vi "MASBstat.vi"() -> ()   [LabVIEW 2020]
doc: "Main application front panel."
uses:
  Typedefs/Control and indicators refs.ctl
  Typedefs/EHL state.ctl
  Global variables/VISA resource.vi
  Global variables/Control and indicators refs.vi
  Typedefs/State.ctl
  Typedefs/CV configuration.ctl
panel:
  out "I-V Graph":cluster{"X":dbl, "Y":dbl}[](graph)
  in  "Connect":bool
  in  "Device":refnum<visa-resource-name>
  in  "Measurement":bool
  in  "CV configuration":T1={"E begin (V)"=0.0, "E vertex 1 (V)"=0.0, "E vertex 2 (V)"=0.0, "Cycles"=1, "Scan rate (V/s)"=0.01, "E step (V)"=0.01} {"E step (V)" min=0.01 max=0.25; "Scan rate (V/s)" min=0.01 max=10.0; "Cycles" min=1; "E vertex 2 (V)" min=-3.3 max=3.3; "E vertex 1 (V)" min=-3.3 max=3.3; "E begin (V)" min=-3.3 max=3.3}
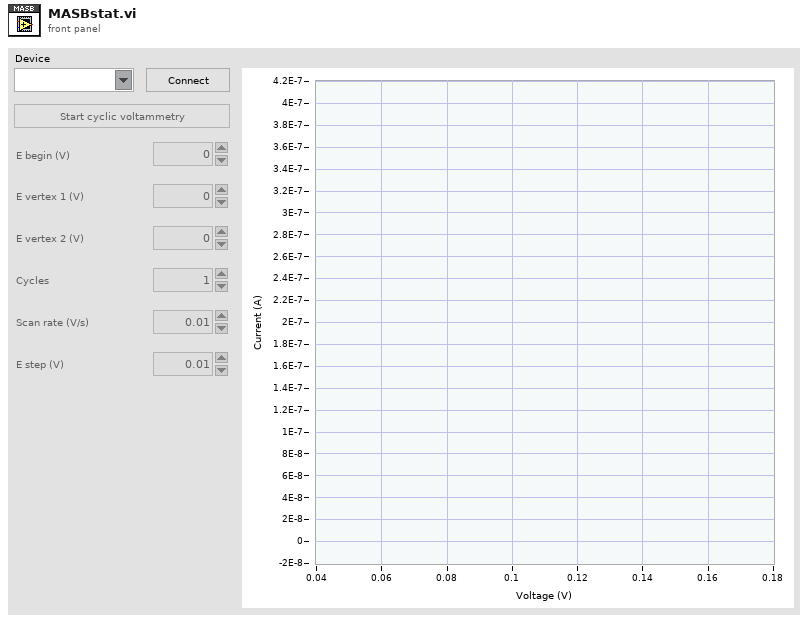
[diagram p1: front panel]
types:
  T1 = typedef "CV configuration.ctl" = cluster{"E begin (V)":dbl, "E vertex 1 (V)":dbl, "E vertex 2 (V)":dbl, "Cycles":u8, "Scan rate (V/s)":dbl, "E step (V)":dbl}
  T2 = typedef "State.ctl" = enum16{"Disconnected", "Connected", "Measuring"}
  T3 = typedef "EHL state.ctl" = cluster{"Semaphore":T4, "Queue":refnum<queue>, "App state":T2}
  T4 = typedef "Semaphore RefNum" = refnum<k1>
  T5 = typedef "Control and indicators refs.ctl" = cluster{"Device":refnum<vi>, "Connect":refnum<vi>, "Measurement":refnum<vi>, "CV configuration":refnum<vi>, "I-V Graph":refnum<vi>}
  T6 = cluster{"E begin (V)":dbl, "E vertex 1 (V)":dbl, "E vertex 2 (V)":dbl, "Cycles":u8, "Scan rate (V/s)":dbl, "E step (V)":dbl}
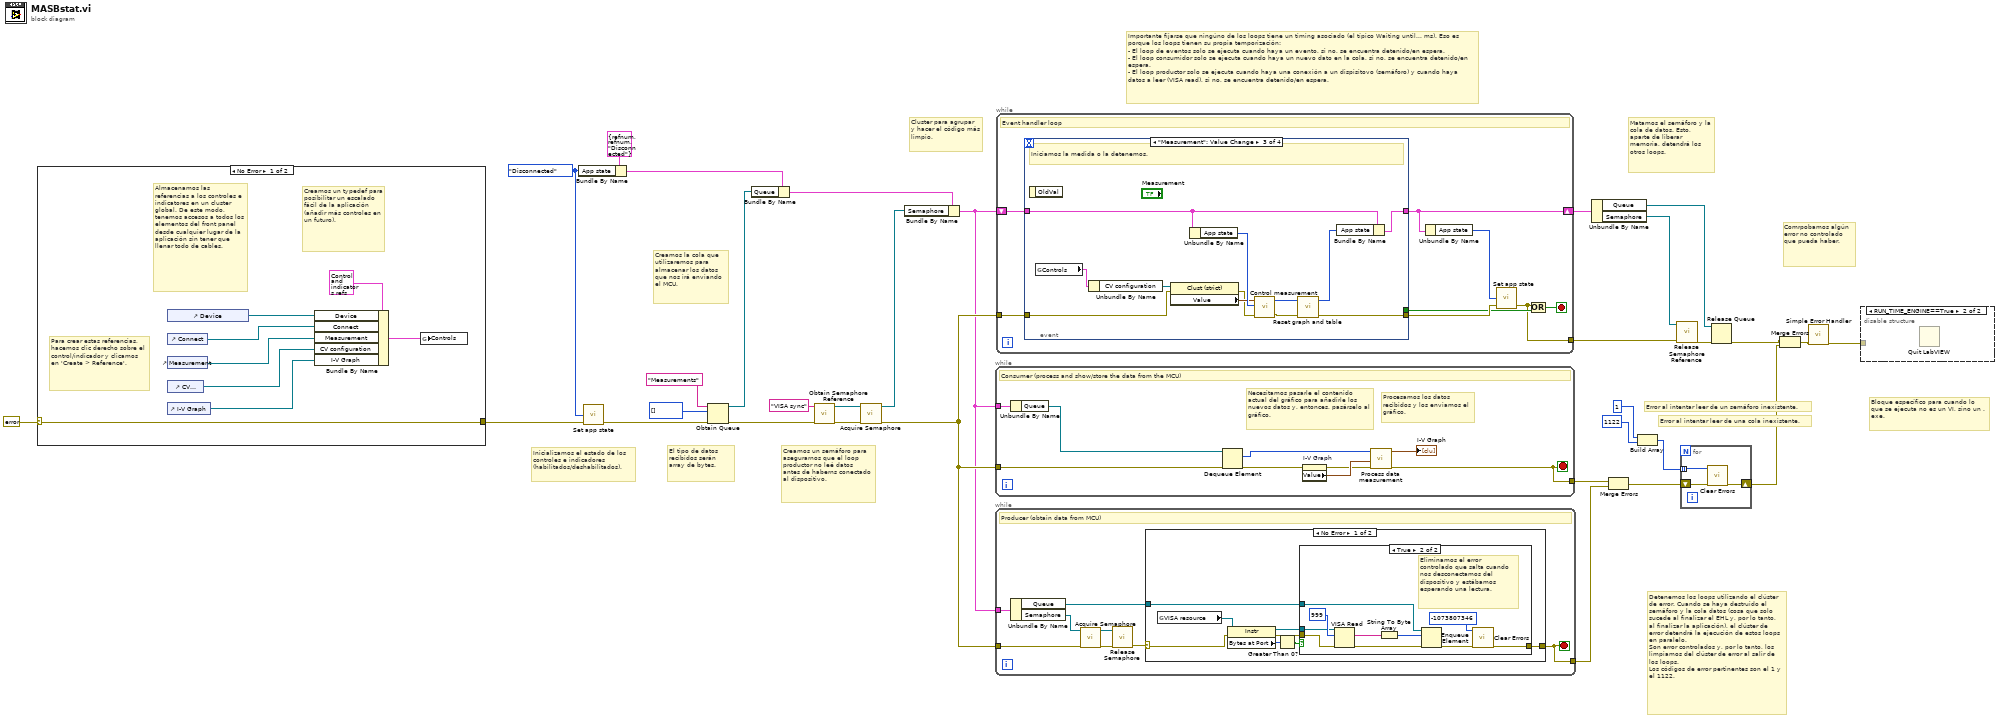
[diagram p0: block diagram]
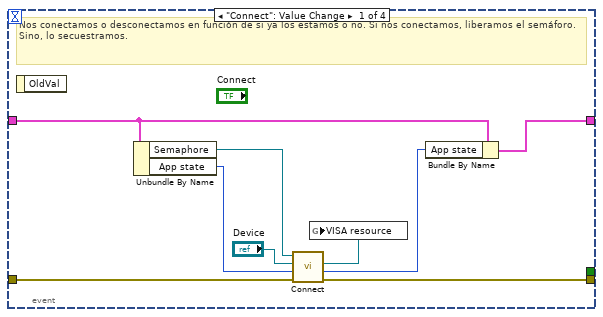
[diagram p4: hidden frame]
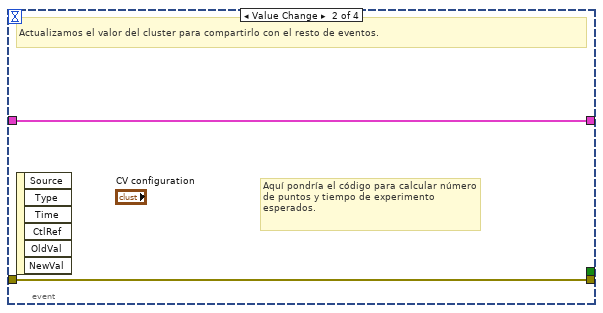
[diagram p5: hidden frame]
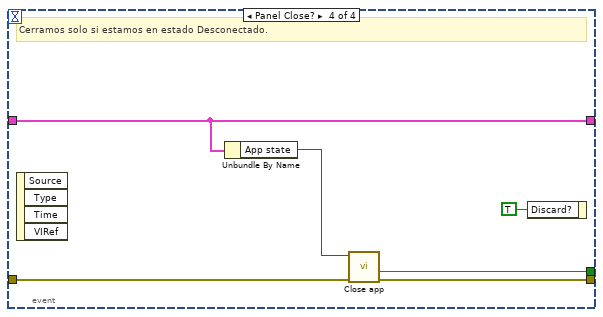
[diagram p6: hidden frame]
diagram:
  w1 = State."Disconnected" ("App state")
  # "Importante fijarse que ningúno de los loops tiene un timing asociado (el típico Waiting until... ms). Eso es porque los loops tienen su propia temporización:\n- El loop de eventos solo se ejecuta cuando haya un evento, si no, se encuentra detenido/en espera.\n- El loop consumidor solo se ejecuta cuando haya un nuevo dato en la cola, si no, se encuentra detenido/en espera.\n- El loop productor solo se ejecuta cuando haya una conexión a un dispisitovo (semáforo) y cuando haya datos a leer (VISA read), si no, se encuentra detenido/en espera."
  # "Bloque específico para cuando lo que se ejecuta no es un VI, sino un .exe."
  # "Comrpobamos algún error no controlado que pueda haber."
  # "Matamos el semáforo y la cola de datos. Esto, aparte de liberar memoria, detendrá los otros loops."
  # "Detenemos los loops utilizando el clúster de error. Cuando se haya destruido el semáforo y la cola datos (cosa que solo sucede al finalizar el EHL y, por lo tanto, al finalizar la aplicación), el clúster de error detendrá la ejecución de estos loops en paralelo.\nSon error controlados y, por lo tanto, los limpiamos del clúster de error al salir de los loops.\nLos códigos de error pertinentes son el 1 y el 1122."
  # "Error al intentar leer de una cola inexistente."
  # "Error al intentar leer de un semáforo inexistente."
  # "Cluster para agrupar y hacer el código más limpio."
  # "Creamos un semáforo para asegurarnos que el loop productor no leé datos antes de haberns conectado al dispositivo."
  # "El tipo de datos recibidos serán array de bytes."
  # "Creamos la cola que utilizaremos para almacenar los datos que nos irá enviando el MCU."
  # "Inicializamos el estado de los controles e indicadores (habilitados/deshabilitados)."
  n1 = case shown="No Error" errorcluster {"status"=FALSE, "code"=0, "source"=""} ("Error in") {
    selector: errorcluster {"status"=FALSE, "code"=0, "source"=""} ("Error in") -> [w34 w41]
    tunnel: [w34 w41] -> w2
    frame No Error {
      # "Creamos un typedef para posibilitar un escalado fácil de la aplicación (añadir más controles en un futuro)."
      # "Para crear estas referencias, hacemos clic derecho sobre el control/indicador y clicamos en 'Create > Reference'."
      # "Almacenamos las referencias a los controles e indicatores en un cluster global. De este modo, tenemos accesos a todos los elementos del front panel desde cualquier lugar de la aplicación sin tener que llenar todo de cables."
      n2 = control-ref of="Device"() -> (w39:refnum<vi>)
      n3 = control-ref of="Connect"() -> (w38:refnum<vi>)
      n4 = control-ref of="Measurement"() -> (w37:refnum<vi>)
      n5 = control-ref of="CV configuration"() -> (w36:refnum<vi>)
      n6 = control-ref of="I-V Graph"() -> (w33:refnum<vi>)
      n7 = Bundle By Name(cluster=T5 {"Device"=refnum, "Connect"=refnum, "Measurement"=refnum, "CV configuration"=refnum, "I-V Graph"=refnum} ("Controls"), "Device"=w39, "Connect"=w38, "Measurement"=w37, "CV configuration"=w36, "I-V Graph"=w33) -> (w35:T5)
      n8 = global write "Control and indicators refs.vi" "Controls"(w35) -> ()
    }
    frame Error {
    }
  }
  n9 = Bundle By Name(cluster=T3 {"Semaphore"=refnum, "Queue"=refnum, "App state"=enum."Disconnected"} ("input cluster"), "App state"=w1) -> (w4:T3)
  n10 = call "Set app state.vi"("Error in"=w2, "App state"=w1) -> ("Error out"=w3:errorcluster)  [unwired: 3 in]
  n11 = Obtain Queue(name (unnamed)="Measurements", element data type=u8[] [] ("Byte array"), error in (no error)=w3) -> (queue out=w19:refnum<queue>, error out=w26:errorcluster)  [unwired: 2 in, 1 out]
  n12 = Bundle By Name(cluster=w4, "Queue"=w19) -> (w18:T3)
  n13 = call <vilib>:"Obtain Semaphore Reference.vi"("error in (no error)"=w26, "name (unnamed)"="VISA sync") -> ("error out"=w27:errorcluster, "semaphore"=w17:T4)  [unwired: 3 in, 1 out]
  n14 = call <vilib>:"Acquire Semaphore.vi"("error in (no error)"=w27, "semaphore"=w17) -> ("error out"=w25:errorcluster, "semaphore out"=w16:T4)  [unwired: 3 in, 1 out]
  n15 = Bundle By Name(cluster=w18, "Semaphore"=w16) -> (w15:T3)
  n16 = while {
    tunnel: w25 -> [w50]
    tunnel: [w47] -> w29
    tunnel: w15 -> [w49]
    stop <- w47 stop-if-true
    # "Necesitamos pasarle el contenido actual del gráfico para añadirle los nuevos datos y, entonces, pasárselo al gráfico."
    # "Procesamos los datos recibidos y los enviamos el gráfico."
    # "Consumer (process and show/store the data from the MCU)"
    n17 = Unbundle By Name(w49) -> ("Queue"=w48:refnum<queue>)
    n18 = Dequeue Element(queue=w48, error in (no error)=w50) -> (element=w42:u8[], error out=w44:errorcluster)  [unwired: 1 in, 2 out]
    n19 = property on="I-V Graph" class="XYGraph (strict)"(error in=w44) -> (error out=w43:errorcluster, "Value"=w45:cluster{"X":dbl, "Y":dbl}[])  [unwired: 1 in, 1 out]
    n20 = call "Process data measurement.vi"("Error in"=w43, "I-V Graph history"=w45, "Byte array"=w42) -> ("Error out"=w47:errorcluster, "I-V Graph"=→"I-V Graph":cluster{"Voltage (V)":dbl, "Current (A)":dbl}[])  [unwired: 7 in]
  }
  n21 = while {
    tunnel: w25 -> [w58]
    tunnel: [w54] -> w28
    tunnel: w15 -> [w57]
    stop <- w54 stop-if-true
    # "Producer (obtain data from MCU)"
    n22 = Unbundle By Name(w57) -> ("Queue"=w56:refnum<queue>, "Semaphore"=w55:T4)
    n23 = call <vilib>:"Acquire Semaphore.vi"("error in (no error)"=w58, "semaphore"=w55) -> ("error out"=w53:errorcluster, "semaphore out"=w52:T4)  [unwired: 3 in, 1 out]
    n24 = call <vilib>:"Release Semaphore.vi"("error in (no error)"=w53, "semaphore"=w52) -> ("error out"=w51:errorcluster)  [unwired: 4 in, 1 out]
    n25 = case shown="No Error" w51 {
      selector: w51 -> [w63 w78]
      tunnel: w56 -> [w66 _]
      tunnel: [w65 w78] -> w54
      frame No Error {
        n26 = global read "VISA resource.vi" "VISA resource"() -> (w64:refnum<visa-resource-name>)
        n27 = property class="Instr"(reference=w64, error in=w63) -> (reference out=w62:refnum<visa-resource-name>, error out=w61:errorcluster, "Bytes at Port"=w60:u32)
        n28 = Greater Than 0?(x=w60) -> (x > 0?=w59:bool)
        n29 = case shown="True" w59 {
          tunnel: w66 -> [_ w74]
          tunnel: [w67 w72] -> w65
          tunnel: w62 -> [_ w69]
          tunnel: w61 -> [w67 w68]
          frame False {
          }
          frame True {
            # "Eliminamos el error controlado que salta cuando nos desconectamos del dispositivo y estábamos esperando una lectura."
            n30 = VISA Read(VISA resource name=w69, byte count=u32 999, error in (no error)=w68) -> (read buffer=w77:string, error out=w75:errorcluster)  [unwired: 2 out]
            n31 = String To Byte Array(string=w77) -> (unsigned byte array=w76:u8[])
            n32 = Enqueue Element(queue=w74, element=w76, error in (no error)=w75) -> (error out=w71:errorcluster)  [unwired: 1 in, 2 out]
            n33 = call <vilib>:"Clear Errors.vi"("error in (no error)"=w71, "specific error code to clear (0: all)"=-1073807346) -> ("error out"=w72:errorcluster)  [unwired: 4 in, 1 out]
          }
        }
      }
      frame Error {
      }
    }
  }
  n34 = while {
    tunnel: w25 -> [w85]
    shift-right: [w80] -> w21
    shift-left: w15 -> [w84]
    tunnel: [w81] -> w7
    stop <- w86 stop-if-true
    # "Event handler loop"
    n35 = event shown="[2] \"Measurement\": Value Change" {
      selector: _ -> [_ _ _ _]
      dyn-events: _ -> [_ _ _ _]
      timeout: _ -> [_ _ _ _]
      tunnel: w85 -> [w90 w97 w98 w110]
      tunnel: [w92 w97 w109 w115] -> w83
      tunnel: [_ _ _ w113] -> w82
      tunnel: w84 -> [w89 w96 w107 w112]
      tunnel: [w87 w96 w106 w112] -> w80
      event "Connect": Value Change {
        # "Nos conectamos o desconectamos en función de si ya los estamos o no. Si nos conectamos, liberamos el semáforo. Sino, lo secuestramos."
        n36 = event-data() -> ()  [unwired: 1 in, 1 out]
        n37 = Unbundle By Name(w89) -> ("Semaphore"=w93:T4, "App state"=w91:T2)
        n38 = call "Connect.vi"("Error in"=w90, "App state"=w91, "VISA resource name"="Device", "Semaphore"=w93) -> ("Error out"=w92:errorcluster, "App state"=w88:T2, "VISA resource name"=w94:refnum<visa-resource-name>)  [unwired: 1 in]
        n39 = global write "VISA resource.vi" "VISA resource"(w94) -> ()
        n40 = Bundle By Name(cluster=w89, "App state"=w88) -> (w87:T3)
      }
      event Value Change {
        # "Aquí pondría el código para calcular número de puntos y tiempo de experimento esperados."
        # "Actualizamos el valor del cluster para compartirlo con el resto de eventos."
        n41 = event-data() -> ()  [unwired: 1 in, 6 out]
      }
      event "Measurement": Value Change {
        # "Iniciamos la medida o la detenemos."
        n42 = event-data() -> ()  [unwired: 1 in, 1 out]
        n43 = global read "Control and indicators refs.vi" "Controls"() -> (w102:T5)
        n44 = Unbundle By Name(w102) -> ("CV configuration"=w101:refnum<vi>)
        n45 = property class="Clust (strict)"(reference=w101, error in=w98) -> (error out=w99:errorcluster, "Value"=w100:T6)  [unwired: 1 out]
        n46 = Unbundle By Name(w107) -> ("App state"=w108:T2)
        n47 = call "Control measurement.vi"("CV configuration"=w100, "App state"=w108, "Error in"=w99) -> ("App state"=w105:T2, "Error out"=w104:errorcluster)  [unwired: 3 in]
        n48 = call "Reset graph and table.vi"("Error in"=w104, "App state"=w105) -> ("Error out"=w109:errorcluster, "App state"=w103:T2)  [unwired: 4 in]
        n49 = Bundle By Name(cluster=w107, "App state"=w103) -> (w106:T3)
      }
      event Panel Close? {
        # "Cerramos solo si estamos en estado Desconectado."
        n50 = event-data() -> ()  [unwired: 1 in, 4 out]
        n51 = Unbundle By Name(w112) -> ("App state"=w111:T2)
        n52 = call "Close app.vi"("Error in"=w110, "App state"=w111) -> ("Error out"=w115:errorcluster, "Close app?"=w113:bool)  [unwired: 7 in, 1 out]
        n53 = event-data("Discard?"=TRUE) -> ()  [unwired: 1 in, 1 out]
      }
    }
    n54 = Unbundle By Name(w80) -> ("App state"=w79:T2)
    n55 = call "Set app state.vi"("Error in"=w83, "App state"=w79) -> ("Error out"=w81:errorcluster)  [unwired: 3 in]
    n56 = Or(x=w81, y=w82) -> (x .or. y?=w86:bool)
  }
  n57 = Unbundle By Name(w21) -> ("Queue"=w14:refnum<queue>, "Semaphore"=w20:T4)
  n58 = Merge Errors(w29, w28) -> (w11:errorcluster)
  n59 = Build Array(1 ("element"), 1122 ("specific error code to clear (0: all)")) -> (w12:i32[])
  n60 = call <vilib>:"Release Semaphore Reference.vi"("error in (no error)"=w7, "semaphore"=w20) -> ("error out"=w23:errorcluster)  [unwired: 8 in, 1 out]
  n61 = for {
    tunnel: w12 -> [w118] mode=indexing
    shift-right: [w116] -> w10
    shift-left: w11 -> [w117]
    n62 = call <vilib>:"Clear Errors.vi"("error in (no error)"=w117, "specific error code to clear (0: all)"=w118) -> ("error out"=w116:errorcluster)  [unwired: 4 in, 1 out]
  }
  n63 = Release Queue(queue=w14, error in (no error)=w23) -> (error out=w22:errorcluster)  [unwired: 1 in, 2 out]
  n64 = Merge Errors(w22, w10) -> (w30:errorcluster)
  n65 = call <vilib>:"Simple Error Handler.vi"("error in (no error)"=w30) -> ("error out"=w32:errorcluster)  [unwired: 4 in, 4 out]
  n66 = disable-structure shown="RUN_TIME_ENGINE==True" {
    disable-tunnel: w32 -> [_ _]
    frame condition #0 (active) {
    }
    frame condition #1 {
      n67 = Quit LabVIEW() -> ()  [unwired: 1 in]
    }
  }
